vi "LabelCaption.vi"(0 "Control in":refnum<vi>) -> (2 "Label.Text":string, 3 "Caption.Text":string, 4 "Tip Strip":string)   [LabVIEW 2021, in "Tree.lvlib" / "Tree.lvclass"]
uses:
  Tree.lvclass
  Tree.lvclass/Tree.ctl
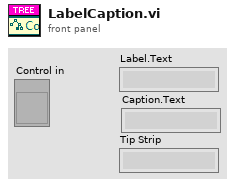
[diagram p1: front panel]
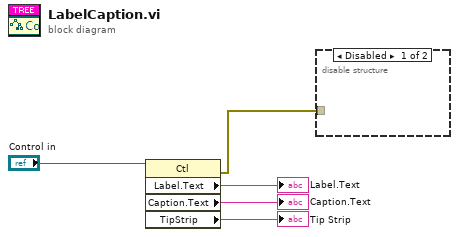
[diagram p0: block diagram]
diagram:
  n1 = property class="Ctl"(reference="Control in") -> (error out=w2:errorcluster, "Label.Text"=→"Label.Text":string, "Caption.Text"=→"Caption.Text":string, "TipStrip"=→"Tip Strip":string)  [unwired: 1 in, 1 out]
  n2 = disable-structure shown="Disabled" {
    disable-tunnel: w2 -> [_ _]
    frame Disabled {
    }
    frame Enabled {
    }
  }
